vi "test_signal_reproduction.vi"() -> ()   [LabVIEW 2020]
uses:
  <vilib>/DAQmx/read.llb/DAQmx Read (Analog 1D DBL 1Chan NSamp).vi
  <vilib>/DAQmx/create/channels.llb/DAQmx Create Channel (AI-Voltage-Basic).vi
  <vilib>/DAQmx/configure/timing.llb/DAQmx Timing (Sample Clock).vi
  <vilib>/DAQmx/miscellaneous.llb/DAQmx Fill In Error Info.vi
  <vilib>/Utility/file.llb/Write Delimited Spreadsheet (DBL).vi
panel:
  in  "scaling ratio (zero for default)":dbl
  in  "Analog out":string(combo)
  out "X":dbl[](array[numeric])
  in  "X file path":path
  in  "Analog in":string(combo)
  out "Analog In Waveform":dbl[](graph)
  in  "save path":path
  in  "rate":dbl
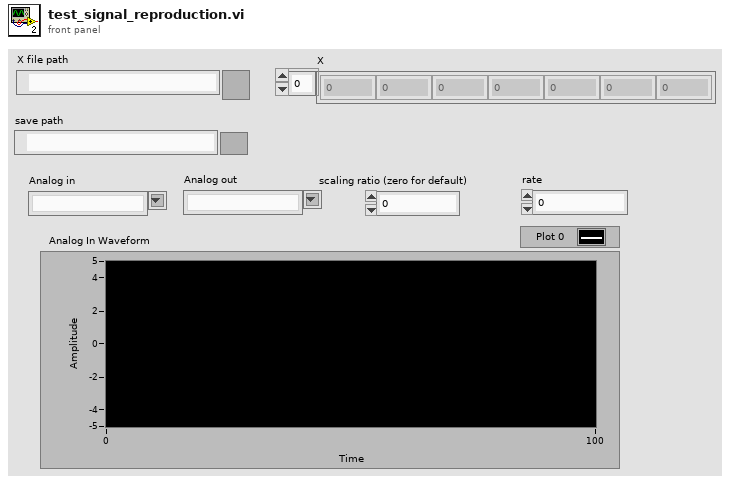
[diagram p1: front panel]
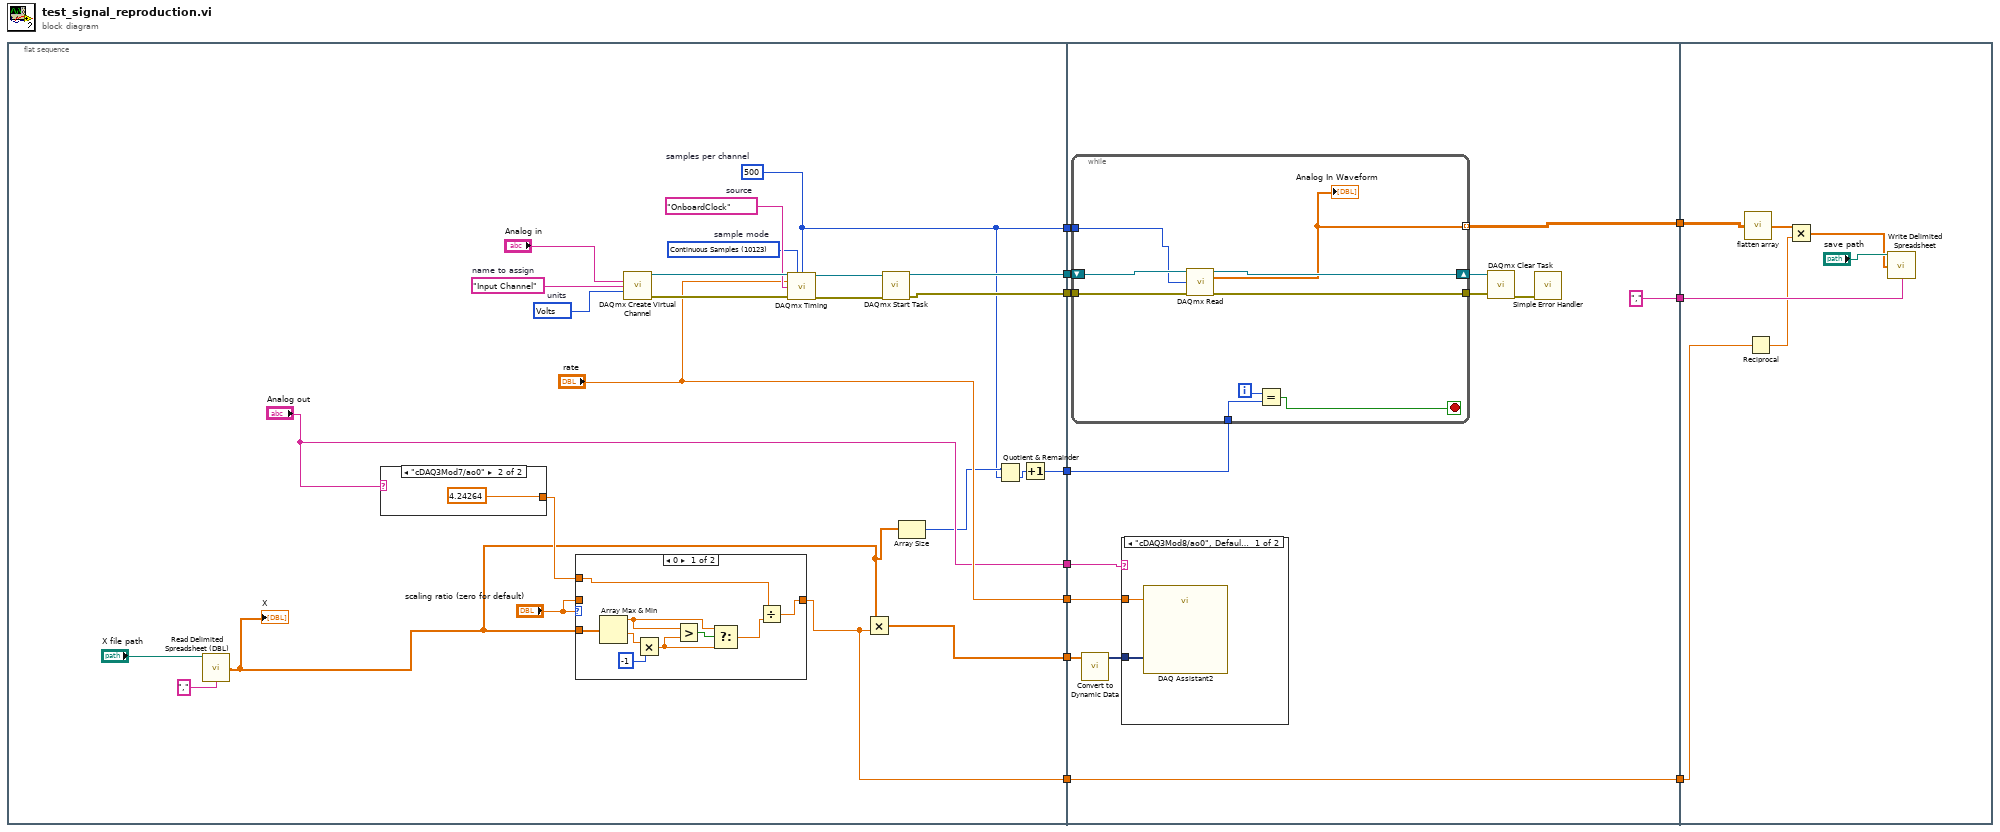
[diagram p0: block diagram]
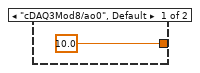
[diagram p2: hidden frame]
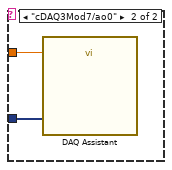
[diagram p4: hidden frame]
diagram:
  n1 = flat-sequence {
    tunnel: [w27] -> w11
    tunnel: [w26] -> w10
    tunnel: ["rate"] -> w9
    tunnel: [w20] -> w8
    tunnel: ["Analog out"] -> w7
    tunnel: [w15] -> w4
    tunnel: [w13] -> w3
    tunnel: [w12] -> w1
    tunnel: w11 -> [w58]
    tunnel: w10 -> [w57]
    tunnel: w9 -> [w56]
    tunnel: w8 -> [w55]
    tunnel: w7 -> [w53]
    tunnel: [w52] -> w6
    tunnel: [","] -> w5
    tunnel: w4 -> [w50]
    tunnel: w3 -> [w49]
    tunnel: [w48] -> w2
    tunnel: w1 -> [w48]
    tunnel: w6 -> [w81]
    tunnel: w5 -> [w80]
    tunnel: w2 -> [w78]
    frame #0 {
      w14 = 10123 items=["Finite Samples"=10178, "Continuous Samples"=10123, "Hardware Timed Single Point"=12522]  # sample mode
      w13 = 500  # samples per channel
      w28 = 10348 items=["Volts"=10348, "From Custom Scale"=10065]  # units
      w32 = tag "OnboardClock"  # source
      w35 = "Input Channel"  # name to assign
      n2 = call <vilib>:"Read Delimited Spreadsheet (DBL).vi"("file path (dialog if empty)"="X file path", "delimiter (\\t)"=",") -> ("first row"=w18:dbl[])  [unwired: 8 in, 5 out]
      "X" <- w18
      n3 = case shown="\"cDAQ3Mod7/ao0\"" "Analog out" {
        tunnel: [10.0 4.24264] -> w22
        frame "cDAQ3Mod8/ao0", Default {
        }
        frame "cDAQ3Mod7/ao0" {
        }
      }
      n4 = case shown="0" "scaling ratio (zero for default)" {
        tunnel: w22 -> [w40 _]
        tunnel: "scaling ratio (zero for default)" -> [_ w47]
        tunnel: [w38 w47] -> w12
        tunnel: w18 -> [w41 _]
        frame 0 {
          n5 = Array Max & Min(array=w41) -> (max value=w44:dbl, min value=w43:dbl)  [unwired: 2 out]
          n6 = Multiply(x=w43, y=-1) -> (x*y=w45:dbl)
          n7 = Greater?(x=w44, y=w45) -> (0:w46:bool)
          n8 = Select(t=w44, s=w46, f=w45) -> (s? t:f=w39:dbl)
          n9 = Divide(x=w40, y=w39) -> (x/y=w38:dbl)
        }
        frame 1, Default {
        }
      }
      n10 = call-poly <vilib>:"DAQmx Create Virtual Channel.vi"("physical channels"="Analog in", "name to assign"=w35, "units"=w28) -> ("task out"=w34:refnum<k21>, "error out"=w33:errorcluster)  [unwired: 11 in]
      n11 = call-poly <vilib>:"DAQmx Timing.vi"("task/channels in"=w34, "sample mode"=w14, "samples per channel"=w13, "rate"="rate", "source"=w32, "error in"=w33) -> ("task out"=w31:refnum<k21>, "error out"=w30:errorcluster)  [unwired: 8 in]
      n12 = Multiply(x=w18, y=w12) -> (x*y=w20:dbl[])
      n13 = call <vilib>:"DAQmx Start Task.vi"("task/channels in"=w31, "error in"=w30) -> ("task out"=w26:refnum<k21>, "error out"=w27:errorcluster)  [unwired: 12 in]
      n14 = Array Size(array=w18) -> (size(s)=w17:i32)
      n15 = Quotient & Remainder(x=w17, y=w13) -> (floor(x/y)=w16:i32)  [unwired: 1 out]
      n16 = Increment(x=w16) -> (x+1=w15:i32)
    }
    frame #1 {
      n17 = while {
        tunnel: w58 -> [w73]
        tunnel: [w71] -> w52 mode=indexing
        shift-right: [w72] -> w60
        shift-left: w57 -> [w74]
        tunnel: [w70] -> w61
        tunnel: w50 -> [w69]
        tunnel: w49 -> [w66]
        i -> [w68]
        stop <- w67 stop-if-true
        n18 = call-poly <vilib>:"DAQmx Read.vi"("task/channels in"=w74, "number of samples per channel"=w66, "error in"=w73) -> ("task out"=w72:refnum<k21>, "data"=w71:dbl[], "error out"=w70:errorcluster)  [unwired: 10 in]
        "Analog In Waveform" <- w71
        n19 = Equal?(x=w68, y=w69) -> (x = y?=w67:bool)
      }
      n20 = call "Convert to Dynamic Data"("Array"=w55) -> ("Dynamic Data Type"=w54:dynamicdata)  [unwired: 3 in]
      n21 = case shown="\"cDAQ3Mod8/ao0\", Default" w53 {
        tunnel: w56 -> [w63 w65]
        tunnel: w54 -> [w62 w64]
        frame "cDAQ3Mod8/ao0", Default {
          n22 = call "DAQ Assistant2"("data"=w62, "rate"=w63) -> ()  [unwired: 15 in, 3 out]
        }
        frame "cDAQ3Mod7/ao0" {
          n23 = call "DAQ Assistant"("data"=w64, "rate"=w65) -> ()  [unwired: 15 in, 3 out]
        }
      }
      n24 = call <vilib>:"DAQmx Clear Task.vi"("task in"=w60, "error in"=w61) -> ("error out"=w59:errorcluster)  [unwired: 13 in]
      n25 = call <vilib>:"Simple Error Handler.vi"("error in (no error)"=w59) -> ()  [unwired: 4 in, 5 out]
    }
    frame #2 {
      n26 = call "flatten array.vi"("in"=w81) -> ("out"=w77:dbl[])
      n27 = Reciprocal(x=w78) -> (1/x=w76:dbl)
      n28 = Multiply(x=w77, y=w76) -> (x*y=w75:dbl[])
      n29 = call-poly <vilib>:"Write Delimited Spreadsheet.vi"("file path (dialog if empty)"="save path", "1D data"=w75, "delimiter (\\t)"=w80) -> ()  [unwired: 11 in, 2 out]
    }
  }
